vi "ErroQuadMedio Calculator.vi"(9 "Sinal original":T1[](array[typedef]) {"height" format="%+4.3f"; "pixel_y" format="%+4.3f"; "pixel_x" format="%+4.3f"; "orientation" format="%+4.3f"; "y" format="%+4.3f"; "confidence" format="%4.3f"; "x" format="%+4.3f"}, 11 "Ruído corrigido":T1[](array[typedef]) {"height" format="%+4.3f"; "pixel_y" format="%+4.3f"; "pixel_x" format="%+4.3f"; "orientation" format="%+4.3f"; "y" format="%+4.3f"; "confidence" format="%4.3f"; "x" format="%+4.3f"}) -> (0 "ErQuadMed Ang_amarelo":sgl, 1 "ErQuadMed Yamarelo":sgl, 2 "ErQuadMed Xamarelo":sgl, 3 "transposed array":sgl[][](array[numeric]), 5 "id order":u32[](array[numeric]))   [LabVIEW 2016]
uses:
  SSL Detection Robot.ctl
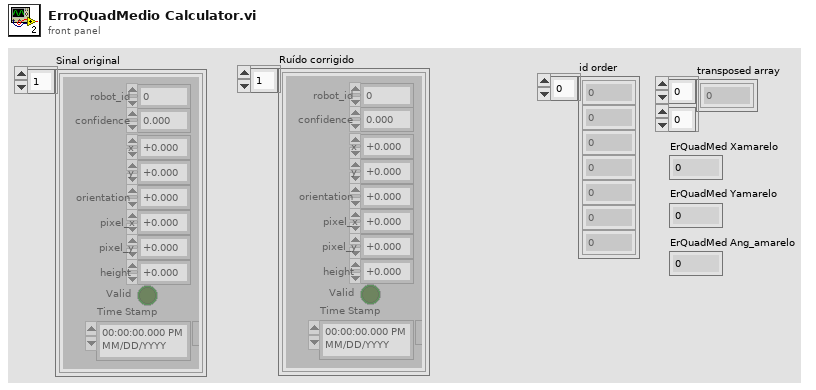
[diagram p1: front panel]
types:
  T1 = typedef "SSL Detection Robot.ctl" = cluster{"x":sgl, "robot_id":u32, "confidence":sgl, "y":sgl, "orientation":sgl, "pixel_x":sgl, "pixel_y":sgl, "height":sgl, "Valid":bool, "Time Stamp":timestamp}
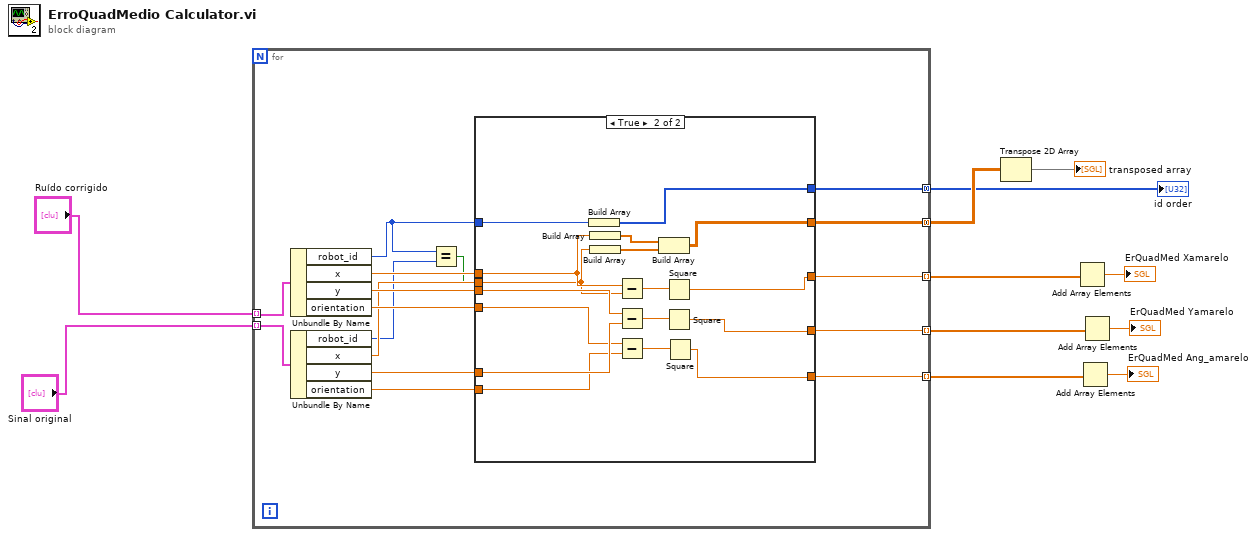
[diagram p0: block diagram]
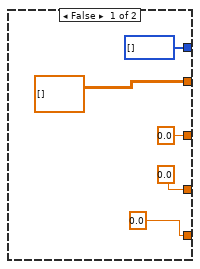
[diagram p2: hidden frame]
diagram:
  n1 = for {
    tunnel: "Ruído corrigido" -> [w27] mode=indexing
    tunnel: "Sinal original" -> [w26] mode=indexing
    tunnel: [w21] -> w3 mode=indexing
    tunnel: [w20] -> w4 mode=indexing
    tunnel: [w19] -> w2 mode=indexing
    tunnel: [w16] -> w11 mode=concatenating
    tunnel: [w15] -> w10 mode=concatenating
    n2 = Unbundle By Name(w27) -> ("robot_id"=w14:u32, "x"=w18:sgl, "y"=w25:sgl, "orientation"=w23:sgl)
    n3 = Unbundle By Name(w26) -> ("robot_id"=w13:u32, "x"=w17:sgl, "y"=w24:sgl, "orientation"=w22:sgl)
    n4 = Equal?(x=w14, y=w13) -> (x = y?=w12:bool)
    n5 = case shown="True" w12 {
      tunnel: w25 -> [_ w49]
      tunnel: w24 -> [_ w48]
      tunnel: w23 -> [_ w47]
      tunnel: w22 -> [_ w46]
      tunnel: [sgl 0.0 w42] -> w21
      tunnel: [sgl 0.0 w41] -> w20
      tunnel: [sgl 0.0 w40] -> w19
      tunnel: w18 -> [_ w39]
      tunnel: w17 -> [_ w37]
      tunnel: [sgl[][] [] w35] -> w16
      tunnel: [u32[] [] w34] -> w15
      tunnel: w14 -> [_ w33]
      frame False {
      }
      frame True {
        n6 = Build Array(w33) -> (w34:u32[])
        n7 = Build Array(w39) -> (w38:sgl[])
        n8 = Build Array(w37) -> (w36:sgl[])
        n9 = Subtract(x=w39, y=w37) -> (x-y=w45:sgl)
        n10 = Subtract(x=w49, y=w48) -> (x-y=w44:sgl)
        n11 = Subtract(x=w47, y=w46) -> (x-y=w43:sgl)
        n12 = Build Array(w38, w36) -> (w35:sgl[][])
        n13 = Square(x=w45) -> (x^2=w42:sgl)
        n14 = Square(x=w44) -> (x^2=w41:sgl)
        n15 = Square(x=w43) -> (x^2=w40:sgl)
      }
    }
  }
  "id order" <- w10
  n16 = Transpose 2D Array(2D array=w11) -> (transposed array=→"transposed array":sgl[][])
  n17 = Add Array Elements(numeric array=w3) -> (sum=→"ErQuadMed Xamarelo":sgl)
  n18 = Add Array Elements(numeric array=w2) -> (sum=→"ErQuadMed Ang_amarelo":sgl)
  n19 = Add Array Elements(numeric array=w4) -> (sum=→"ErQuadMed Yamarelo":sgl)
